vi "Untitledn.vi"() -> ()   [LabVIEW 2023]
panel:
  out "element":string
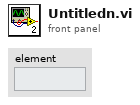
[diagram p1: front panel]
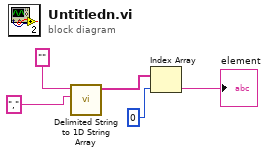
[diagram p0: block diagram]
diagram:
  n1 = call <vilib>:"Delimited String to 1D String Array.vi"("delimiter"=",", "delimited string"="") -> ("string array"=w4:string[])  [unwired: 9 in]
  n2 = Index Array(array=w4, index=0) -> (element=→"element":string)
